vi "PLCControl.vi"() -> ()   [LabVIEW 2017]
uses:
  <vilib>/NI/Modbus Library/API/Wrapper/Create TCP Master.vi
  <vilib>/NI/Modbus Library/API/Master/Modbus Master.lvclass
  <vilib>/NI/Modbus Library/API/Wrapper/API Main.lvlib
panel:
  out "Time":dbl
  in  "Set Zero Speed":bool
  in  "Time (min)":dbl format="%#_13g"
  in  "Timing Exp":bool
  in  "stop":bool
  out "Applied":i32
  out "AntiClockWise 2":bool
  out "Nplc 2":i32
  in  "AntiClockWise":bool
  out "x-y":i32[](array[numeric])
  out "32bit integer 2":i32[](array[numeric])
  out "T Exp (min)":dbl
  out "RPM":dbl
  out "T Exp (min)":dbl
  out "Linear Speed (microns/min)":dbl
  in  "Nplc":dbl=1000000.0
  in  "Nplc Set":u32
  out "T Exp Set Ro t (min)":dbl
  out "T Exp Set Lin (min)":dbl
  out "Nplc Lin Set":u32
  in  "Select Linear Speed \n(microns/s)":dbl=1.0
  in  "Select RPM":dbl=0.12
  out "Nplc Rot Sel":u32
  out "microns/min Lin":dbl
  out "RPM Rot":dbl
  out "Nplc Rot":u32
  out "Nplc Lin":u32
  in  "T Exp (min)":dbl=60.0
  in  "Check":bool
  out "microns/min":dbl
  out "RPM":dbl
  in  "Np":dbl=1000000.0
  in  "Write":bool
  in  "Read":bool
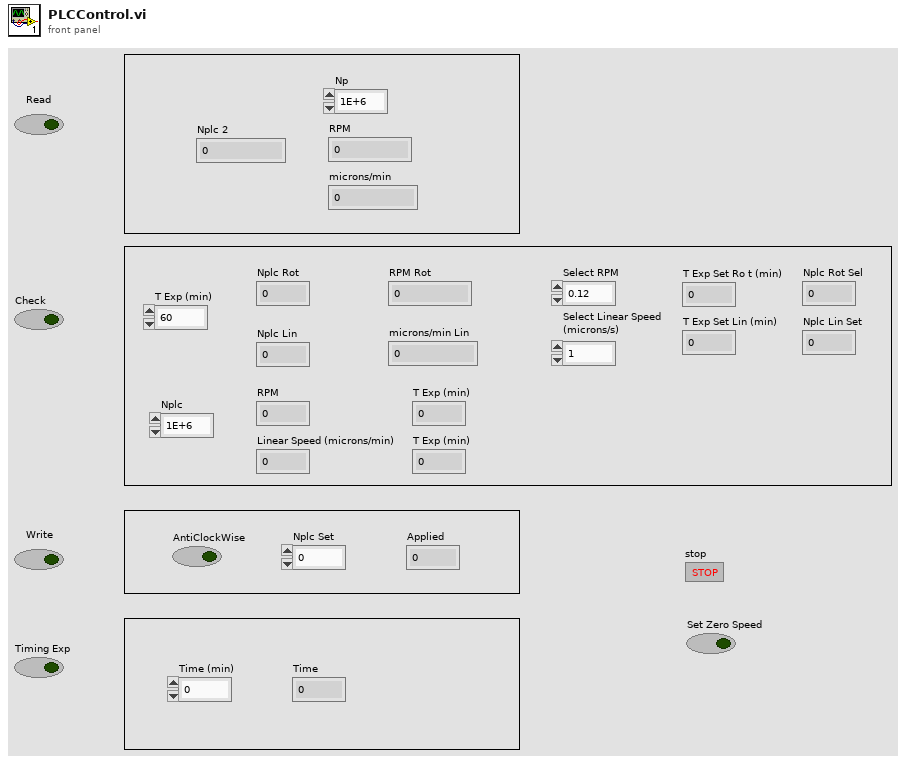
[diagram p1: front panel]
types:
  T1 = cluster{"[0]":u16, "[1]":u16, "[2]":u16, "[3]":u16, "[4]":u16, "[5]":u16, "[6]":u16, "[7]":u16, "[8]":u16}
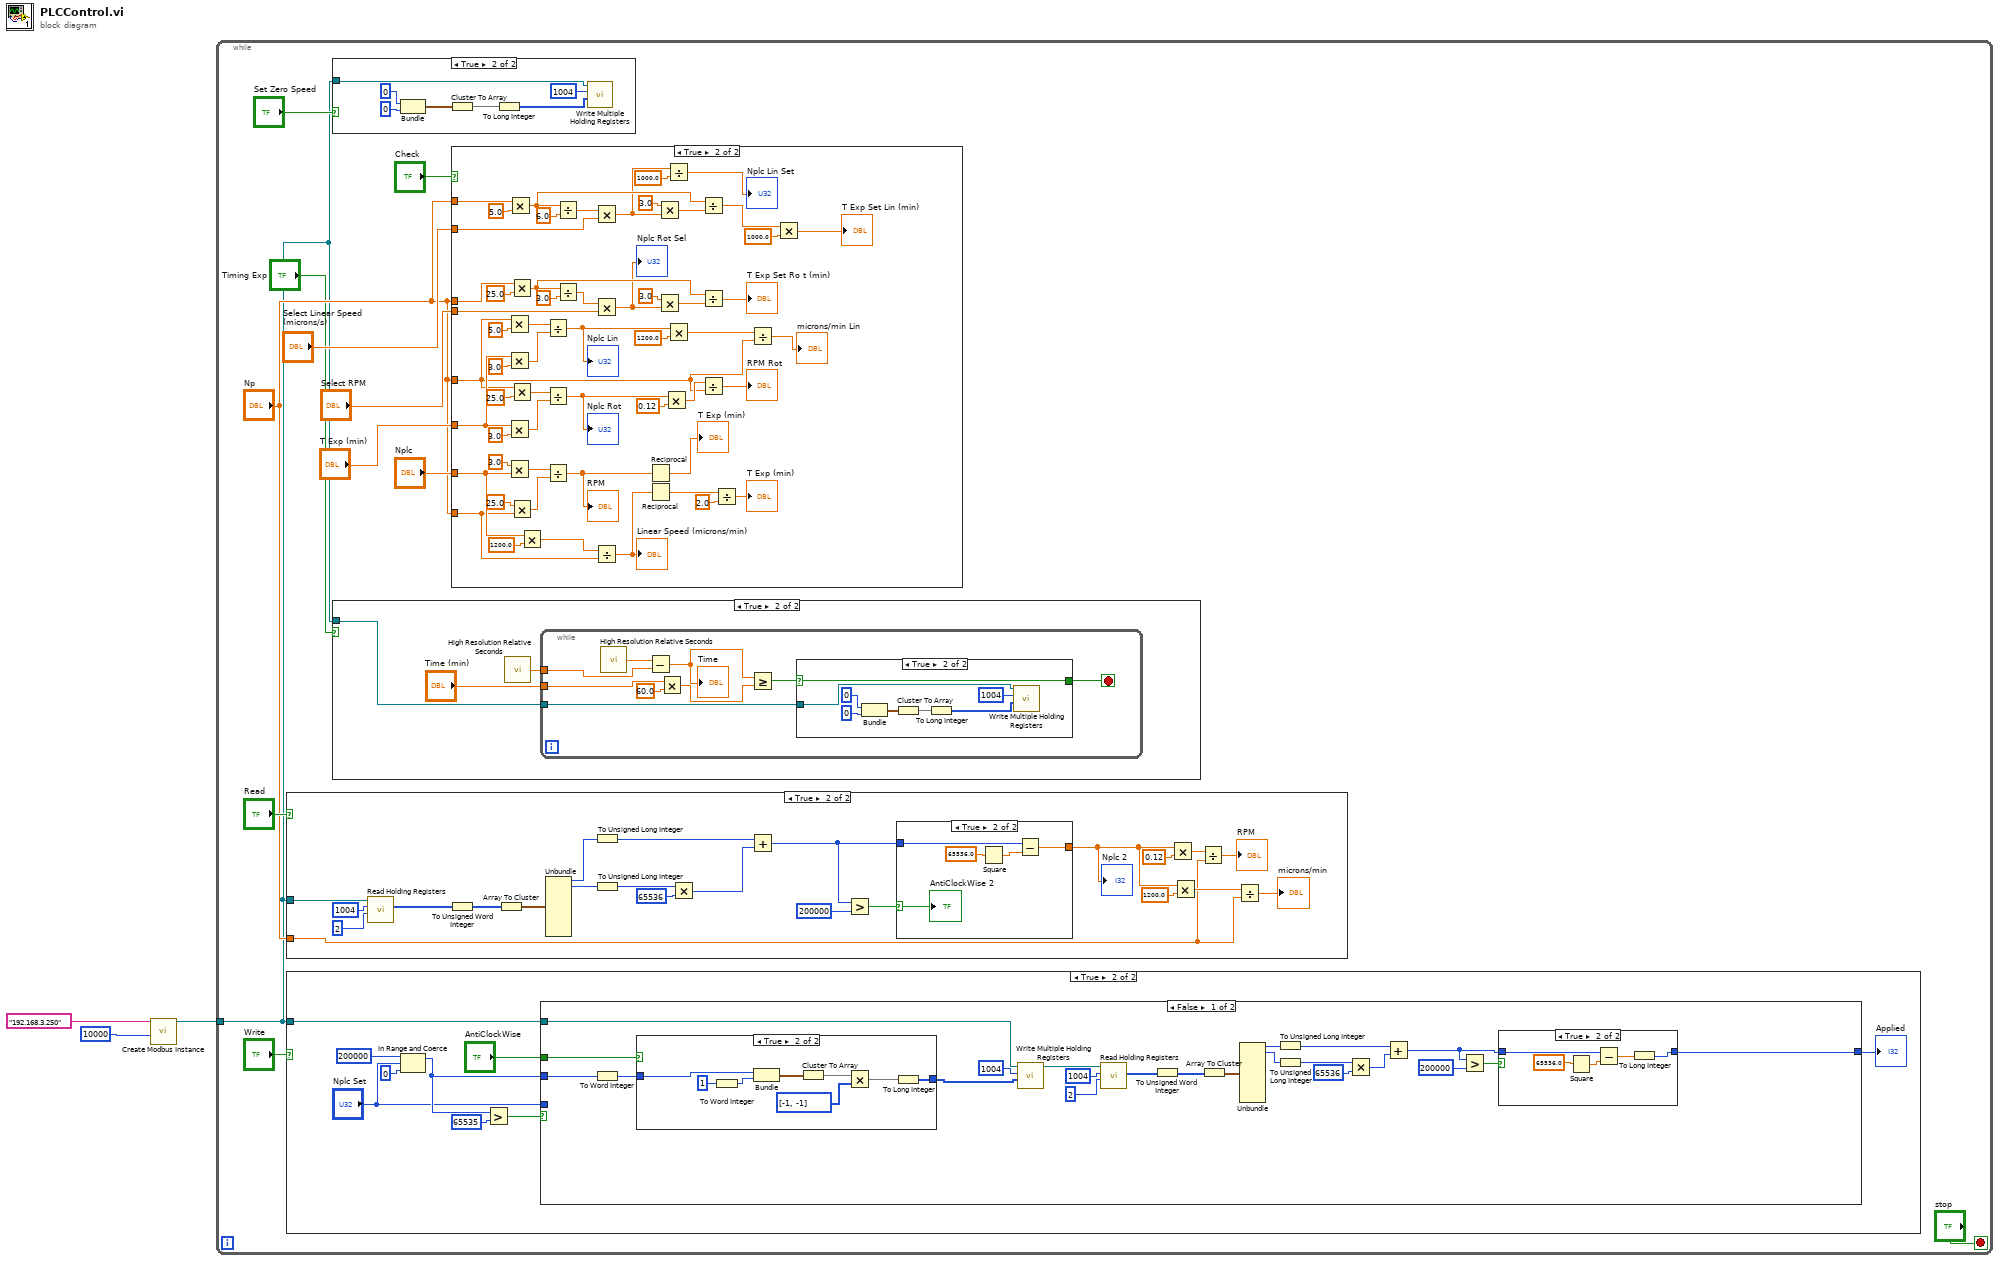
[diagram p0: block diagram]
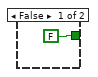
[diagram p4: hidden frame]
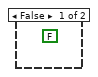
[diagram p6: hidden frame]
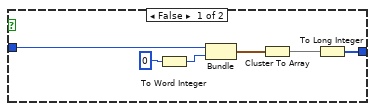
[diagram p8: hidden frame]
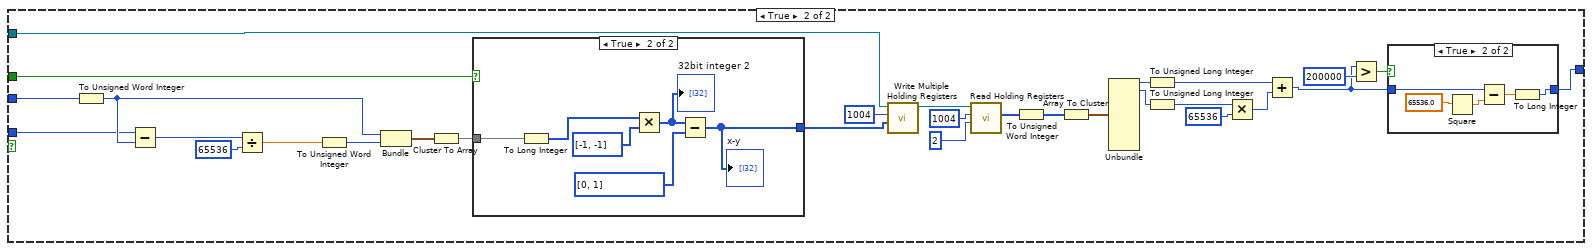
[diagram p9: hidden frame]
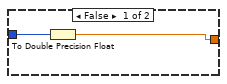
[diagram p13: hidden frame]
diagram:
  n1 = call-poly <vilib>:"Create Modbus Instance.vi"("connect timeout ms"=10000, "address"="192.168.3.250") -> ("TCP master instance"=w1:refnum<class "Modbus Master.lvclass">)  [unwired: 8 in, 1 out]
  n2 = while {
    tunnel: w1 -> [w4]
    stop <- "stop" stop-if-true
    n3 = case shown="True" "Read" {
      tunnel: w4 -> [_ w196]
      tunnel: "Np" -> [_ w202]
      frame False {
      }
      frame True {
        n4 = call-dynamic "Read Holding Registers.vi"("number of inputs"=u16 2, "starting address"=u16 1004, "Modbus master in"=w196) -> ("register values"=w193:u16[])  [unwired: 6 in, 2 out]
        n5 = To Unsigned Word Integer(number=w193) -> (unsigned 16bit integer=w201:u16[])
        n6 = Array To Cluster(array=w201) -> (cluster=w213:T1)
        n7 = Unbundle(w213) -> ("[0]"=w208:u16, "[1]"=w195:u16)  [unwired: 7 out]
        n8 = To Unsigned Long Integer(number=w208) -> (unsigned 32bit integer=w207:u32)
        n9 = To Unsigned Long Integer(number=w195) -> (unsigned 32bit integer=w194:u32)
        n10 = Multiply(x=w194, y=u32 65536) -> (x*y=w211:u32)
        n11 = Add(x=w207, y=w211) -> (x+y=w198:u32)
        n12 = Greater?(x=w198, y=u32 200000) -> (0:w199:bool)
        n13 = case shown="True" w199 {
          selector: w199 -> [_ w218]
          tunnel: w198 -> [w217 w222]
          tunnel: [w216 w219] -> w197
          frame False {
            n14 = To Double Precision Float(number=w217) -> (double precision float=w216:dbl)
          }
          frame True {
            n15 = Square(x=65536.0) -> (x^2=w221:dbl)
            n16 = Subtract(x=w222, y=w221) -> (x-y=w219:dbl)
            "AntiClockWise 2" <- w218
          }
        }
        "Nplc 2" <- w197
        n17 = Multiply(x=w197, y=0.12) -> (x*y=w210:dbl)
        n18 = Multiply(x=w197, y=1200.0) -> (x*y=w206:dbl)
        n19 = Divide(x=w210, y=w202) -> (x/y=→"RPM":dbl)
        n20 = Divide(x=w206, y=w202) -> (x/y=→"microns/min":dbl)
      }
    }
    n21 = case shown="True" "Write" {
      tunnel: w4 -> [_ w103]
      frame False {
        (unwired) FALSE
      }
      frame True {
        n22 = In Range and Coerce(upper limit=u32 200000, x="Nplc Set", lower limit=u32 0) -> (coerced(x)=w106:u32)  [unwired: 1 out]
        n23 = Greater?(x=w106, y=u32 65535) -> (0:w104:bool)
        n24 = case shown="False" w104 {
          tunnel: w106 -> [w130 w179]
          tunnel: w103 -> [w128 w172]
          tunnel: "AntiClockWise" -> [w127 w168]
          tunnel: [w111 w152] -> w101
          tunnel: "Nplc Set" -> [_ w151]
          frame False {
            n25 = To Word Integer(number=w130) -> (16bit integer=w109:i16)
            n26 = case shown="True" w127 {
              tunnel: w109 -> [w139 w144]
              tunnel: [w137 w148] -> w110
              frame False {
                n27 = To Word Integer(number=i16 0) -> (16bit integer=w142:i16)
                n28 = Bundle(w139, w142) -> (w141:cluster{i16, i16})  [unwired: 1 in]
                n29 = Cluster To Array(cluster=w141) -> (array=w138:i16[])
                n30 = To Long Integer(number=w138) -> (32bit integer=w137:i32[])
              }
              frame True {
                n31 = To Word Integer(number=i16 1) -> (16bit integer=w147:i16)
                n32 = Bundle(w144, w147) -> (w146:cluster{i16, i16})  [unwired: 1 in]
                n33 = Cluster To Array(cluster=w146) -> (array=w143:i16[])
                n34 = Multiply(x=w143, y=i16[] [-1, -1]) -> (x*y=w149:i16[])
                n35 = To Long Integer(number=w149) -> (32bit integer=w148:i32[])
              }
            }
            n36 = call-dynamic "Write Multiple Holding Registers.vi"("registers to write"=w110, "starting address"=u16 1004, "Modbus master in"=w128) -> ("Modbus master out"=w112:refnum<class "Modbus Master.lvclass">)  [unwired: 7 in, 1 out]
            n37 = call-dynamic "Read Holding Registers.vi"("number of inputs"=u16 2, "starting address"=u16 1004, "Modbus master in"=w112) -> ("register values"=w113:u16[])  [unwired: 6 in, 2 out]
            n38 = To Unsigned Word Integer(number=w113) -> (unsigned 16bit integer=w119:u16[])
            n39 = Array To Cluster(array=w119) -> (cluster=w124:T1)
            n40 = Unbundle(w124) -> ("[0]"=w121:u16, "[1]"=w115:u16)  [unwired: 7 out]
            n41 = To Unsigned Long Integer(number=w121) -> (unsigned 32bit integer=w120:u32)
            n42 = To Unsigned Long Integer(number=w115) -> (unsigned 32bit integer=w114:u32)
            n43 = Multiply(x=w114, y=u32 65536) -> (x*y=w122:u32)
            n44 = Add(x=w120, y=w122) -> (x+y=w116:u32)
            n45 = Greater?(x=w116, y=u32 200000) -> (0:w117:bool)
            n46 = case shown="True" w117 {
              tunnel: w116 -> [w131 w136]
              tunnel: [w131 w132] -> w111
              frame False {
              }
              frame True {
                n47 = Square(x=65536.0) -> (x^2=w135:dbl)
                n48 = Subtract(x=w136, y=w135) -> (x-y=w133:dbl)
                n49 = To Long Integer(number=w133) -> (32bit integer=w132:i32)
              }
            }
          }
          frame True {
            n50 = To Unsigned Word Integer(number=w179) -> (unsigned 16bit integer=w174:u16)
            n51 = Subtract(x=w151, y=w174) -> (x-y=w178:u32)
            n52 = Divide(x=w178, y=u32 65536) -> (x/y=w176:dbl)
            n53 = To Unsigned Word Integer(number=w176) -> (unsigned 16bit integer=w175:u16)
            n54 = Bundle(w174, w175) -> (w173:cluster{u16, u16})  [unwired: 1 in]
            n55 = Cluster To Array(cluster=w173) -> (array=w170:u16[])
            n56 = case shown="True" w168 {
              tunnel: w170 -> [w186 w192]
              tunnel: [w186 w187] -> w169
              frame False {
              }
              frame True {
                n57 = To Long Integer(number=w192) -> (32bit integer=w191:i32[])
                n58 = Multiply(x=w191, y=i32[] [-1, -1]) -> (x*y=w189:i32[])
                "32bit integer 2" <- w189
                n59 = Subtract(x=w189, y=i32[] [0, 1]) -> (x-y=w187:i32[])
                "x-y" <- w187
              }
            }
            n60 = call-dynamic "Write Multiple Holding Registers.vi"("registers to write"=w169, "starting address"=u16 1004, "Modbus master in"=w172) -> ("Modbus master out"=w153:refnum<class "Modbus Master.lvclass">)  [unwired: 7 in, 1 out]
            n61 = call-dynamic "Read Holding Registers.vi"("number of inputs"=u16 2, "starting address"=u16 1004, "Modbus master in"=w153) -> ("register values"=w154:u16[])  [unwired: 6 in, 2 out]
            n62 = To Unsigned Word Integer(number=w154) -> (unsigned 16bit integer=w160:u16[])
            n63 = Array To Cluster(array=w160) -> (cluster=w165:T1)
            n64 = Unbundle(w165) -> ("[0]"=w162:u16, "[1]"=w156:u16)  [unwired: 7 out]
            n65 = To Unsigned Long Integer(number=w162) -> (unsigned 32bit integer=w161:u32)
            n66 = To Unsigned Long Integer(number=w156) -> (unsigned 32bit integer=w155:u32)
            n67 = Multiply(x=w155, y=u32 65536) -> (x*y=w163:u32)
            n68 = Add(x=w161, y=w163) -> (x+y=w157:u32)
            n69 = Greater?(x=w157, y=u32 200000) -> (0:w158:bool)
            n70 = case shown="True" w158 {
              tunnel: w157 -> [w180 w185]
              tunnel: [w180 w181] -> w152
              frame False {
              }
              frame True {
                n71 = Square(x=65536.0) -> (x^2=w184:dbl)
                n72 = Subtract(x=w185, y=w184) -> (x-y=w182:dbl)
                n73 = To Long Integer(number=w182) -> (32bit integer=w181:i32)
              }
            }
          }
        }
        "Applied" <- w101
      }
    }
    n74 = case shown="True" "Set Zero Speed" {
      tunnel: w4 -> [_ w16]
      frame False {
      }
      frame True {
        n75 = Bundle(i16 0, i16 0) -> (w19:cluster{i16, i16})  [unwired: 1 in]
        n76 = Cluster To Array(cluster=w19) -> (array=w18:i16[])
        n77 = To Long Integer(number=w18) -> (32bit integer=w17:i32[])
        n78 = call-dynamic "Write Multiple Holding Registers.vi"("registers to write"=w17, "starting address"=u16 1004, "Modbus master in"=w16) -> ()  [unwired: 7 in, 2 out]
      }
    }
    n79 = case shown="True" "Timing Exp" {
      tunnel: w4 -> [_ w23]
      frame False {
      }
      frame True {
        n80 = call <vilib>:"High Resolution Relative Seconds.vi"() -> ("relative seconds"=w25:dbl)
        n81 = while {
          tunnel: w25 -> [w33]
          tunnel: "Time (min)" -> [w30]
          tunnel: w23 -> [w27]
          stop <- w26 stop-if-true
          n82 = call <vilib>:"High Resolution Relative Seconds.vi"() -> ("relative seconds"=w34:dbl)
          n83 = Subtract(x=w34, y=w33) -> (x-y=w32:dbl)
          "Time" <- w32
          n84 = Multiply(x=w30, y=60.0) -> (x*y=w29:dbl)
          n85 = Greater Or Equal?(x=w32, y=w29) -> (x >= y?=w28:bool)
          n86 = case shown="True" w28 {
            selector: w28 -> [_ w36]
            tunnel: w27 -> [_ w37]
            tunnel: [FALSE w36] -> w26
            frame False {
            }
            frame True {
              n87 = Bundle(i16 0, i16 0) -> (w40:cluster{i16, i16})  [unwired: 1 in]
              n88 = Cluster To Array(cluster=w40) -> (array=w39:i16[])
              n89 = To Long Integer(number=w39) -> (32bit integer=w38:i32[])
              n90 = call-dynamic "Write Multiple Holding Registers.vi"("registers to write"=w38, "starting address"=u16 1004, "Modbus master in"=w37) -> ()  [unwired: 7 in, 2 out]
            }
          }
        }
      }
    }
    n91 = case shown="True" "Check" {
      tunnel: "Np" -> [_ w84]
      tunnel: "T Exp (min)" -> [_ w91]
      tunnel: "Np" -> [_ w79]
      tunnel: "Select RPM" -> [_ w78]
      tunnel: "Select Linear Speed \n(microns/s)" -> [_ w72]
      tunnel: "Np" -> [_ w74]
      tunnel: "Nplc" -> [_ w51]
      tunnel: "Np" -> [_ w48]
      frame False {
      }
      frame True {
        n92 = Multiply(x=w84, y=5.0) -> (x*y=w97:dbl)
        n93 = Multiply(x=w91, y=3.0) -> (x*y=w96:dbl)
        n94 = Multiply(x=w91, y=3.0) -> (x*y=w92:dbl)
        n95 = Multiply(x=3.0, y=w51) -> (x*y=w47:dbl)
        n96 = Multiply(x=w74, y=5.0) -> (x*y=w71:dbl)
        n97 = Multiply(x=w79, y=25.0) -> (x*y=w68:dbl)
        n98 = Multiply(x=w84, y=25.0) -> (x*y=w93:dbl)
        n99 = Multiply(x=25.0, y=w48) -> (x*y=w46:dbl)
        n100 = Multiply(x=w51, y=1200.0) -> (x*y=w56:dbl)
        n101 = Divide(x=w97, y=w96) -> (x/y=w82:dbl)
        "Nplc Lin" <- w82
        n102 = Divide(x=w93, y=w92) -> (x/y=w83:dbl)
        "Nplc Rot" <- w83
        n103 = Divide(x=w47, y=w46) -> (x/y=w45:dbl)
        "RPM" <- w45
        n104 = Divide(x=w71, y=6.0) -> (x/y=w73:dbl)
        n105 = Divide(x=w68, y=3.0) -> (x/y=w77:dbl)
        n106 = Multiply(x=w73, y=w72) -> (x*y=w60:dbl)
        n107 = Multiply(x=w77, y=w78) -> (x*y=w65:dbl)
        "Nplc Rot Sel" <- w65
        n108 = Divide(x=w56, y=w48) -> (x/y=w55:dbl)
        "Linear Speed (microns/min)" <- w55
        n109 = Reciprocal(x=w45) -> (1/x=→"T Exp (min)":dbl)
        n110 = Reciprocal(x=w55) -> (1/x=w54:dbl)
        n111 = Multiply(x=3.0 ("y"), y=w60) -> (x*y=w69:dbl)
        n112 = Multiply(x=3.0, y=w65) -> (x*y=w67:dbl)
        n113 = Multiply(x=w83, y=0.12) -> (x*y=w90:dbl)
        n114 = Divide(x=w60, y=1000.0) -> (x/y=→"Nplc Lin Set":dbl)
        n115 = Multiply(x=w82, y=1200.0) -> (x*y=w88:dbl)
        n116 = Divide(x=w71, y=w69) -> (x/y=w62:dbl)
        n117 = Divide(x=w68, y=w67) -> (x/y=→"T Exp Set Ro t (min)":dbl)
        n118 = Divide(x=w90, y=w84) -> (x/y=→"RPM Rot":dbl)
        n119 = Divide(x=w54, y=2.0) -> (x/y=→"T Exp (min)":dbl)
        n120 = Divide(x=w88, y=w84) -> (x/y=→"microns/min Lin":dbl)
        n121 = Multiply(x=w62, y=1000.0) -> (x*y=→"T Exp Set Lin (min)":dbl)
      }
    }
  }
